vi "ISX3_Cmd_SetSetupInit.vi"() -> (0 "set Setup Init Cmd":u8[](array[numeric]))   [LabVIEW 2012, in "Sciospec ISX3 Impedance Analyzer.lvlib"]
uses:
  Sciospec ISX3 Impedance Analyzer.lvlib
panel:
  # "This VI generates the command initate a new setup in the system.\nAny previous setting are cleared."
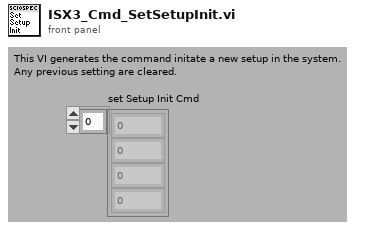
[diagram p1: front panel]
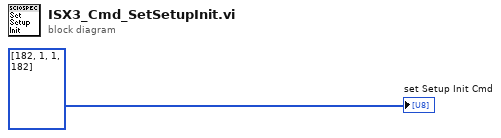
[diagram p0: block diagram]
diagram:
  "set Setup Init Cmd" <- u8[] [182, 1, 1, 182]
